vi "solving_linear_equation_function(SubVI).vi"(10 "Wektor b":dbl[](array[numeric]), 11 "Macierz A":dbl[][](array[numeric])) -> (3 "Wynik":dbl[](array[numeric]))   [LabVIEW 2020]
uses:
  <vilib>/Analysis/7linalg.llb/Solve Linear Equations (single right hand).vi
  <vilib>/Analysis/baseanly.llb/Solve Linear Equations By Cholesky.vi
  <vilib>/Analysis/baseanly.llb/Real Matrix to Compact Array.vi
  <vilib>/Analysis/baseanly.llb/Real Compact Tri-Matrix Linear Eqs.vi
  <vilib>/Analysis/7linalg.llb/Solve Linear Eqs (General).vi
  <vilib>/Analysis/7linalg.llb/Solve Linear Eqs (Gen, single right hand).vi
  <vilib>/Analysis/NI_AALPro.lvlib
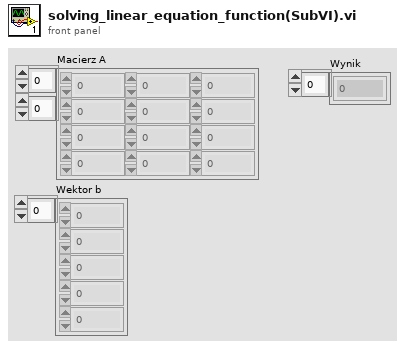
[diagram p1: front panel]
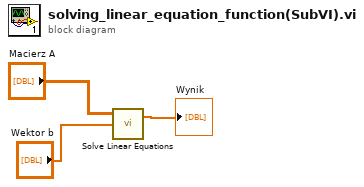
[diagram p0: block diagram]
diagram:
  n1 = call-poly <vilib>:"Solve Linear Equations.vi"("Known Vector"="Wektor b", "Input Matrix"="Macierz A") -> ("Solution Vector"=→"Wynik":dbl[])  [unwired: 1 in, 1 out]
